vi "daqmx frequency trial.vi"   [LabVIEW 2018]
uses:
  <vilib>/DAQmx/create/channels.llb/DAQmx Create Channel (CI-Frequency).vi
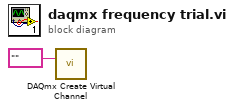
[diagram p0: block diagram]
diagram:
  n1 = call-poly <vilib>:"DAQmx Create Virtual Channel.vi"("counter"=tag "") -> ()  [unwired: 13 in, 2 out]
